vi "Init.vi"(8 "error in (no error)":errorcluster, 10 "Address":string, 11 "DongWoo.lvlib:DongWoo.lvclass":refnum<class "DongWoo.lvclass">) -> (0 "error out":errorcluster, 3 "DongWoo.lvlib:DongWoo.lvclass":refnum<class "DongWoo.lvclass">)   [LabVIEW 2023, in "DongWoo_Spectrometer.lvlib" / "DongWoo.lvclass"]
uses:
  DongWoo.lvclass
  DongWoo.lvclass/DongWoo.ctl
  <vilib>/ActorFramework/Actor/Actor.lvclass/Actor.ctl
  Interfaces/InitDeinitInterface/InitDeinitComm Messages/InitDone Msg/InitDone Msg.lvclass/InitDone Msg.ctl
  <vilib>/ActorFramework/Message Enqueuer/Message Enqueuer.lvclass/Message Enqueuer.ctl
  <vilib>/ActorFramework/Message Enqueuer/Enqueue.vi
  Interfaces/InitDeinitInterface/InitDeinitComm Messages/InitDone Msg/InitDone Msg.lvclass
  <vilib>/Instr/_visa.llb/VISA Configure Serial Port (Instr).vi
  <vilib>/Utility/LVClass/Get LV Class Name.vi
  <resource>/AFDebug/Generate Trace for Message.vi
  <vilib>/ActorFramework/Message Priority Queue/Priority Enqueue.vi
  <vilib>/ActorFramework/Actor/Actor.lvclass
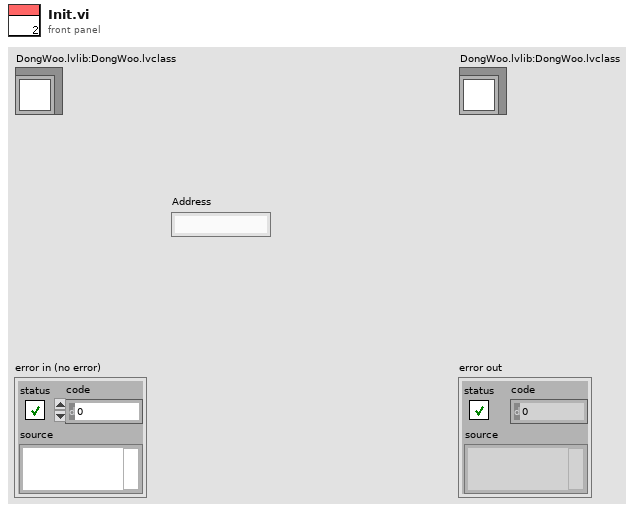
[diagram p1: front panel]
types:
  T1 = typedef "typedefs.lvlib/instrumentType.ctl" = enum16{"Spectrum Analyzer", "Spectrometer", "Camera", "Stepper", "Piezo", "SLM"}
  T2 = cluster{"address type":enum16{"VISA", "Index"}, "Address":string, "instrument type":T1}
  T3 = typedef "typedefs.lvlib/SpectroData.ctl" = cluster{"Wavelength":dbl, "Grating":u8, "Entrance ":enum16{"FRONT", "SIDE"}, "Exit ":enum16{"FRONT", "SIDE"}, "Entrance Front Slitwidth":u16, "Entrance Side Slitwidth":u16, "Exit Front Slitwidth":u16, "Exit Side Slitwidth":u16, "Brand":enum16{"HRS", "Dongwoo"}, "Trace Enabled":bool}
  T4 = cluster{"Instr Error":errorcluster, "Address":cluster{"address type":enum16{"VISA", "Index"}, "Address":string, "instrument type":T1}, "SpectroData":T3}
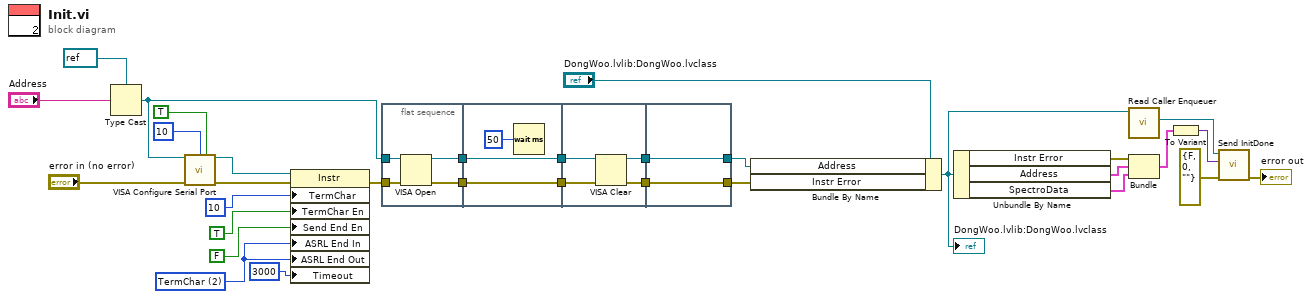
[diagram p0: block diagram]
diagram:
  w13 = u16 2 items=["None", "Last Bit", "TermChar"] ("Serial Settings:End Mode for Reads")
  n1 = Type Cast(type=refnum<visa-resource-name> refnum ("VISA resource name"), x="Address") -> (*(type *) &x=w17:refnum<visa-resource-name>)
  n2 = call-poly "VISA Configure Serial Port"("VISA resource name"=w17, "termination char\n(0xA = '\\n' = LF)"=u8 10 ("Message Based Settings:Termination Character"), "Enable Termination\nChar (T)"=TRUE ("Enable Termination\nChar (T)"), "error in (no error)"="error in (no error)") -> ("VISA resource name out"=w12:refnum<visa-resource-name>, "error out"=w11:errorcluster)  [unwired: 10 in]
  n3 = property class="Instr"(reference=w12, error in=w11, "TermChar"=u8 10 ("Message Based Settings:Termination Character"), "TermChar En"=TRUE ("Message Based Settings:Termination Character Enable"), "Send End En"=FALSE ("Message Based Settings:Send End Enable"), "ASRL End In"=w13, "ASRL End Out"=w13, "Timeout"=u32 3000 ("General Settings:Timeout Value")) -> (error out=w10:errorcluster)  [unwired: 1 out]
  n4 = flat-sequence {
    tunnel: w17 -> [w36]
    tunnel: w10 -> [w35]
    tunnel: [w34] -> w32
    tunnel: [w33] -> w31
    tunnel: w32 -> [w38]
    tunnel: [w38] -> w30
    tunnel: w31 -> [w37]
    tunnel: [w37] -> w29
    tunnel: w30 -> [w43]
    tunnel: w29 -> [w42]
    tunnel: [w41] -> w28
    tunnel: [w40] -> w27
    tunnel: [w44] -> w25
    tunnel: [w45] -> w24
    tunnel: w28 -> [w45]
    tunnel: w27 -> [w44]
    frame #0 {
      n5 = VISA Open(error in (no error)=w35, VISA resource name=w36) -> (VISA resource name=w34:refnum<visa-resource-name>, error out=w33:errorcluster)  [unwired: 3 in]
    }
    frame #1 {
      n6 = Wait (ms)(milliseconds to wait=u32 50) -> ()  [unwired: 1 out]
    }
    frame #2 {
      n7 = VISA Clear(VISA resource name=w43, error in (no error)=w42) -> (VISA resource name out=w40:refnum<visa-resource-name>, error out=w41:errorcluster)
    }
    frame #3 {
    }
  }
  n8 = Bundle By Name(cluster="DongWoo.lvlib:DongWoo.lvclass", "Address"=w25, "Instr Error"=w24) -> (w1:refnum<class "DongWoo.lvclass">)
  "DongWoo.lvlib:DongWoo.lvclass" <- w1
  n9 = Unbundle By Name(w1) -> ("Instr Error"=w21:errorcluster, "Address"=w20:T2, "SpectroData"=w22:T3)
  n10 = call <vilib>:"Read Caller Enqueuer.vi"("Actor"=w1) -> ("Caller Enqueuer"=w2:refnum<class "Message Enqueuer.lvclass">)  [unwired: 10 in]
  n11 = Bundle("Instr Error"=w21, "Address"=w20, "SpectroData"=w22) -> (w19:T4)  [unwired: 1 in]
  n12 = To Variant(anything=w19) -> (Variant=w18:variant)
  n13 = call "Send InitDone.vi"("error in (no error)"=errorcluster {"status"=FALSE, "code"=0, "source"=""}, "Variant"=w18, "Message Enqueuer"=w2) -> ("error out"=→"error out":errorcluster)  [unwired: 7 in, 1 out]
